vi "Encode GND Parameters.vi"(6 "Internal Scanner Exists?":bool=TRUE, 8 "ADD Parameters (in)":string, 9 "VISA resource name":refnum<visa-resource-name>, 10 "Scanner Channel (0 - 16) (0=Off)":u32, 11 "GND Test Paramameters":T1={"Current (1 - 32 A) (25A)"=25.0, "Voltage (3 - 8 V) (8V)"=8.0, "High Limit (0 - 200 mohm)(100 mohm)"=100, "Low Limit (0 - 200 mohm)(0 mohm)"=0, "High Limit V (0 - 6.00 V) (6V)"=6.0, "Low Limit V (0 - 6.00 V) (0V)"=0.0, "Dwell Time (0.0, 0.5 - 999.9 s) (1.0S)"=1.0, "Offset (0 - 200 mohm) (0mohm)"=0, "Offset V (0 - 6.00 V) (0V)"=0.0, "Frequency (50/60 HZ) (50HZ)"=enum."50", "Auto Offset (F: Off)"=FALSE} {"Offset V (0 - 6.00 V) (0V)" format="%#.2f"; "Dwell Time (0.0, 0.5 - 999.9 s) (1.0S)" format="%.1f"; "Low Limit V (0 - 6.00 V) (0V)" format="%#.2f"; "High Limit V (0 - 6.00 V) (6V)" format="%#.2f"; "Voltage (3 - 8 V) (8V)" format="%.2f"; "Current (1 - 32 A) (25A)" format="%.2f"}) -> (1 "Scanner Channel out":u32, 2 "GND Test Paramameters out":T1={"Current (1 - 32 A) (25A)"=25.0, "Voltage (3 - 8 V) (8V)"=8.0, "High Limit (0 - 200 mohm)(100 mohm)"=100, "Low Limit (0 - 200 mohm)(0 mohm)"=0, "High Limit V (0 - 6.00 V) (6V)"=6.0, "Low Limit V (0 - 6.00 V) (0V)"=0.0, "Dwell Time (0.0, 0.5 - 999.9 s) (1.0S)"=1.0, "Offset (0 - 200 mohm) (0mohm)"=0, "Offset V (0 - 6.00 V) (0V)"=0.0, "Frequency (50/60 HZ) (50HZ)"=enum."50", "Auto Offset (F: Off)"=FALSE} {"Offset V (0 - 6.00 V) (0V)" format="%#.2f"; "Dwell Time (0.0, 0.5 - 999.9 s) (1.0S)" format="%.1f"; "Low Limit V (0 - 6.00 V) (0V)" format="%#.2f"; "High Limit V (0 - 6.00 V) (6V)" format="%#.2f"; "Voltage (3 - 8 V) (8V)" format="%.2f"; "Current (1 - 32 A) (25A)" format="%.2f"}, 3 "Add Step":string)   [LabVIEW 2020, in "Associated Research 78XX Series.lvlib"]
uses:
  <instrlib>/Associated Research 78XX Series/Associated Research 78XX Series.lvlib
  <instrlib>/Associated Research 78XX Series/Public/Configure/Steps/Low Level/GND Test Parameters.ctl
panel:
  # "NOTE:\nFirmware version greater than 2.00.00, the following parameters are workable.\nHigh Limit V (0 - 6.00 V)\nLow Limit V (0 - 6.00 V)\nOffset V (0 - 6.00 V)"
  # "On\nOff"
  # "On\nOff"
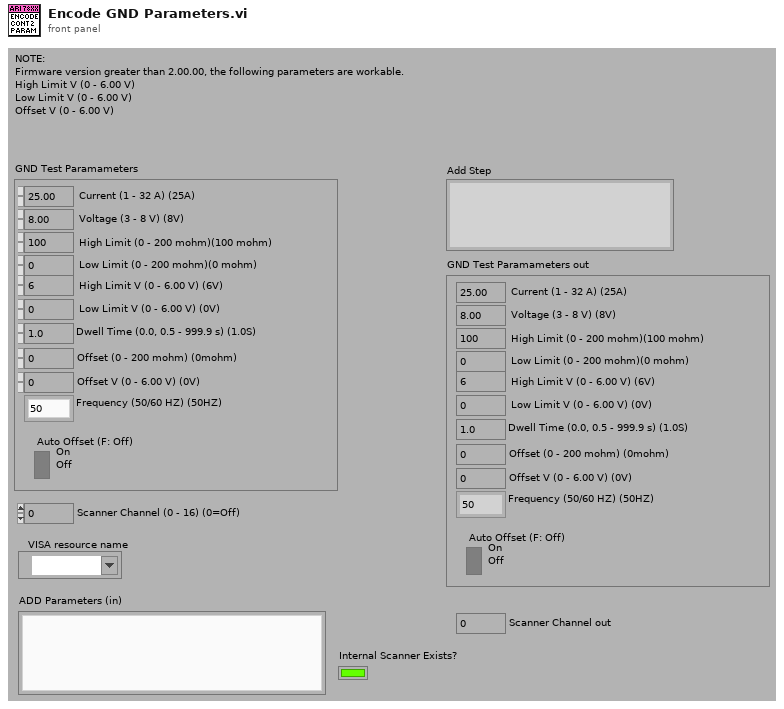
[diagram p1: front panel]
types:
  T1 = typedef "Associated Research 78XX Series.lvlib/GND Test Parameters.ctl" = cluster{"Current (1 - 32 A) (25A)":dbl, "Voltage (3 - 8 V) (8V)":dbl, "High Limit (0 - 200 mohm)(100 mohm)":i32, "Low Limit (0 - 200 mohm)(0 mohm)":i32, "High Limit V (0 - 6.00 V) (6V)":dbl, "Low Limit V (0 - 6.00 V) (0V)":dbl, "Dwell Time (0.0, 0.5 - 999.9 s) (1.0S)":dbl, "Offset (0 - 200 mohm) (0mohm)":i32, "Offset V (0 - 6.00 V) (0V)":dbl, "Frequency (50/60 HZ) (50HZ)":enum16{"50", "60"}, "Auto Offset (F: Off)":bool}
  T2 = typedef "Associated Research 78XX Series.lvlib/Extended User Data.ctl" = cluster{"Firmware Version":string, "Ultra Models":enum16{"7800", "7804", "7820", "7850", "7854"}}
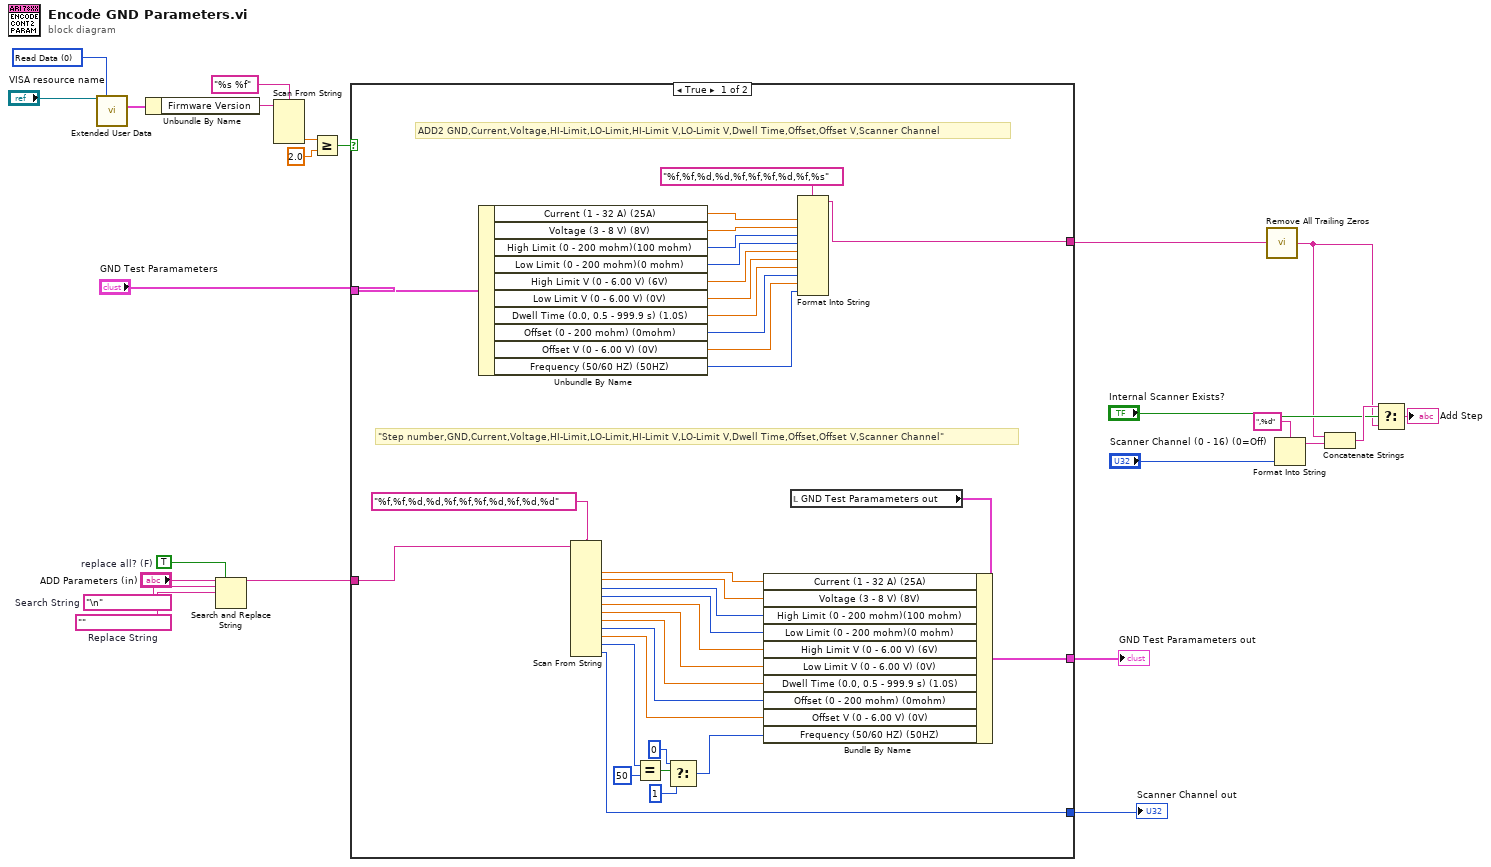
[diagram p0: block diagram]
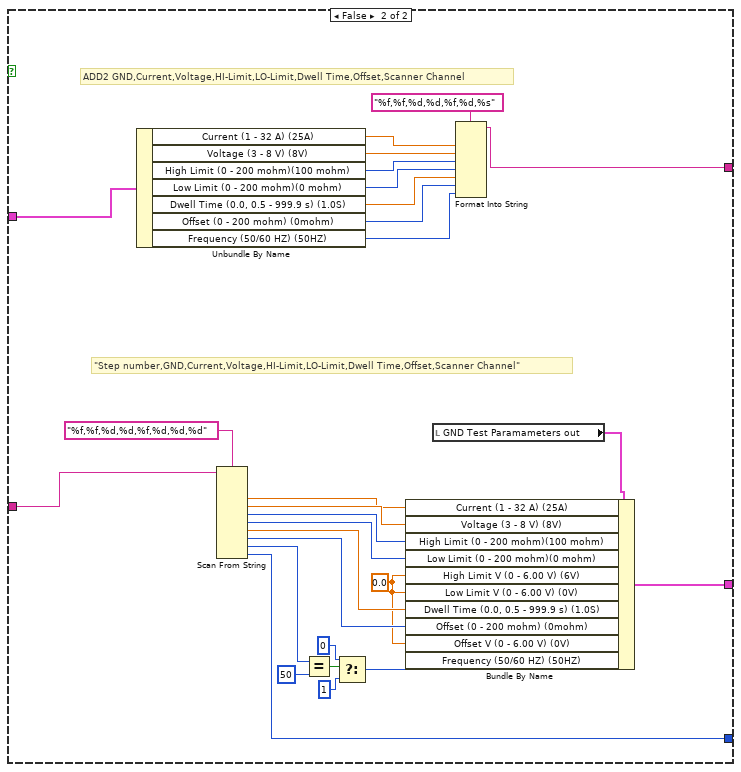
[diagram p2: hidden frame]
diagram:
  w5 = u16 0 items=["Read Data", "Write Data", "Clear Data", "Clear ALL Data"] ("Action")
  w21 = TRUE  # replace all? (F)
  w22 = ""  # Replace String
  w23 = "\n"  # Search String
  n1 = call <instrlib>:"Extended User Data.vi"("VISA resource name"="VISA resource name", "Action"=w5) -> ("User Data Out"=w7:T2)  [unwired: 11 in, 2 out]
  n2 = Unbundle By Name(w7) -> ("Firmware Version"=w12:string)
  n3 = Search and Replace String(replace all?=w21, input string="ADD Parameters (in)", search string=w23, replace string=w22) -> (result string=w3:string)  [unwired: 4 in, 3 out]
  n4 = Scan From String(format string="%s %f", input string=w12) -> (output 2=w10:dbl)  [unwired: 5 in, 3 out]
  n5 = Greater Or Equal?(x=w10, y=2.0) -> (x >= y?=w8:bool)
  n6 = case shown="True" w8 {
    tunnel: [w45 w76] -> w14
    tunnel: "GND Test Paramameters" -> [w50 w78]
    tunnel: w3 -> [w28 w66]
    tunnel: [w27 w59] -> w2
    tunnel: [w26 w61] -> w1
    frame True {
      # "\"Step number,GND,Current,Voltage,HI-Limit,LO-Limit,HI-Limit V,LO-Limit V,Dwell Time,Offset,Offset V,Scanner Channel\""
      # "ADD2 GND,Current,Voltage,HI-Limit,LO-Limit,HI-Limit V,LO-Limit V,Dwell Time,Offset,Offset V,Scanner Channel"
      n7 = Unbundle By Name(w50) -> ("Current (1 - 32 A) (25A)"=w54:dbl, "Voltage (3 - 8 V) (8V)"=w55:dbl, "High Limit (0 - 200 mohm)(100 mohm)"=w56:i32, "Low Limit (0 - 200 mohm)(0 mohm)"=w57:i32, "High Limit V (0 - 6.00 V) (6V)"=w48:dbl, "Low Limit V (0 - 6.00 V) (0V)"=w47:dbl, "Dwell Time (0.0, 0.5 - 999.9 s) (1.0S)"=w52:dbl, "Offset (0 - 200 mohm) (0mohm)"=w51:i32, "Offset V (0 - 6.00 V) (0V)"=w46:dbl, "Frequency (50/60 HZ) (50HZ)"=w49:enum16{"50", "60"})
      n8 = Scan From String(format string="%f,%f,%d,%d,%f,%f,%f,%d,%f,%d,%d" ("Format String"), input string=w28) -> (output 1=w29:dbl, output 2=w30:dbl, output 3=w31:i32, output 4=w32:i32, output 5=w42:dbl, output 6=w43:dbl, output 7=w33:dbl, output 8=w34:i32, output 9=w44:dbl, output 10=w40:i32, output 11=w26:i32)  [unwired: 13 in, 3 out]
      n9 = Equal?(x=w40, y=50) -> (x = y?=w36:bool)
      n10 = Select(t=0, s=w36, f=1) -> (s? t:f=w41:i32)
      n11 = local read "GND Test Paramameters out"() -> (w38:T1)
      n12 = Bundle By Name(cluster=w38, "Current (1 - 32 A) (25A)"=w29, "Voltage (3 - 8 V) (8V)"=w30, "High Limit (0 - 200 mohm)(100 mohm)"=w31, "Low Limit (0 - 200 mohm)(0 mohm)"=w32, "High Limit V (0 - 6.00 V) (6V)"=w42, "Low Limit V (0 - 6.00 V) (0V)"=w43, "Dwell Time (0.0, 0.5 - 999.9 s) (1.0S)"=w33, "Offset (0 - 200 mohm) (0mohm)"=w34, "Offset V (0 - 6.00 V) (0V)"=w44, "Frequency (50/60 HZ) (50HZ)"=w41) -> (w27:T1)
      n13 = Format Into String(format string="%f,%f,%d,%d,%f,%f,%f,%d,%f,%s" ("Format String"), w54, w55, w56, w57, w48, w47, w52, w51, w46, w49) -> (resulting string=w45:string)  [unwired: 2 in, 1 out]
    }
    frame False {
      w60 = 0.0 ("High Limit V (0 - 6.00 V) (6V)")
      # "\"Step number,GND,Current,Voltage,HI-Limit,LO-Limit,Dwell Time,Offset,Scanner Channel\""
      # "ADD2 GND,Current,Voltage,HI-Limit,LO-Limit,Dwell Time,Offset,Scanner Channel"
      n14 = Unbundle By Name(w78) -> ("Current (1 - 32 A) (25A)"=w82:dbl, "Voltage (3 - 8 V) (8V)"=w83:dbl, "High Limit (0 - 200 mohm)(100 mohm)"=w84:i32, "Low Limit (0 - 200 mohm)(0 mohm)"=w85:i32, "Dwell Time (0.0, 0.5 - 999.9 s) (1.0S)"=w80:dbl, "Offset (0 - 200 mohm) (0mohm)"=w79:i32, "Frequency (50/60 HZ) (50HZ)"=w77:enum16{"50", "60"})
      n15 = Scan From String(format string="%f,%f,%d,%d,%f,%d,%d,%d" ("Format String"), input string=w66) -> (output 1=w67:dbl, output 2=w68:dbl, output 3=w69:i32, output 4=w70:i32, output 5=w65:dbl, output 6=w63:i32, output 7=w62:i32, output 8=w61:i32)  [unwired: 10 in, 3 out]
      n16 = Equal?(x=w62, y=50) -> (x = y?=w71:bool)
      n17 = Select(t=0, s=w71, f=1) -> (s? t:f=w75:i32)
      n18 = local read "GND Test Paramameters out"() -> (w74:T1)
      n19 = Bundle By Name(cluster=w74, "Current (1 - 32 A) (25A)"=w67, "Voltage (3 - 8 V) (8V)"=w68, "High Limit (0 - 200 mohm)(100 mohm)"=w69, "Low Limit (0 - 200 mohm)(0 mohm)"=w70, "High Limit V (0 - 6.00 V) (6V)"=w60, "Low Limit V (0 - 6.00 V) (0V)"=w60, "Dwell Time (0.0, 0.5 - 999.9 s) (1.0S)"=w65, "Offset (0 - 200 mohm) (0mohm)"=w63, "Offset V (0 - 6.00 V) (0V)"=w60, "Frequency (50/60 HZ) (50HZ)"=w75) -> (w59:T1)
      n20 = Format Into String(format string="%f,%f,%d,%d,%f,%d,%s" ("Format String"), w82, w83, w84, w85, w80, w79, w77) -> (resulting string=w76:string)  [unwired: 2 in, 1 out]
    }
  }
  "Scanner Channel out" <- w1
  "GND Test Paramameters out" <- w2
  n21 = call <instrlib>:"Remove All Trailing Zeros.vi"("String in"=w14) -> ("String out"=w13:string)
  n22 = Format Into String(format string=",%d" ("Format String"), "Scanner Channel (0 - 16) (0=Off)") -> (resulting string=w4:string)  [unwired: 2 in, 1 out]
  n23 = Concatenate Strings(w13, w4) -> (w24:string)
  n24 = Select(t=w24, s="Internal Scanner Exists?", f=w13) -> (s? t:f=→"Add Step":string)
